vi "DAQ- Steper 2.vi"(0 "Travel (Degree)":dbl=100.0, 5 "Mode":i32(ring)=10178 items=["Finite Samples"=10178, "Continuous Samples"=10123, "Hardware Timed Single Point"=12522], 7 "Home Done":bool, 9 "Speed d/s":dbl=10.0, 11 "error in":errorcluster) -> (6 "Task Done Bit":bool, 15 "error out":errorcluster)   [LabVIEW 2015]
uses:
  Project Setup/Globle Variable/GR_Servo.vi
  <vilib>/DAQmx/create/channels.llb/DAQmx Create Channel (CO-Pulse Generation-Frequency).vi
  <vilib>/DAQmx/configure/timing.llb/DAQmx Timing (Implicit).vi
  Galobal variable_TI.vi
panel:
  out "32bit integer":i32
  in  "Motor PPR":dbl=3600.0
  in  "Motor Gear Ratio":dbl=1.0
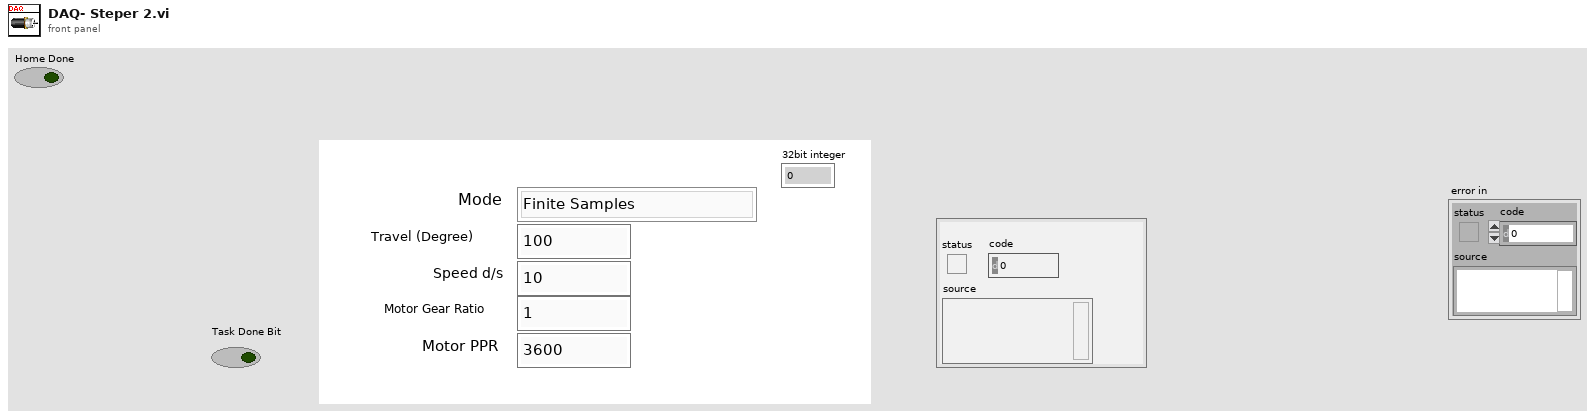
[diagram p1: front panel]
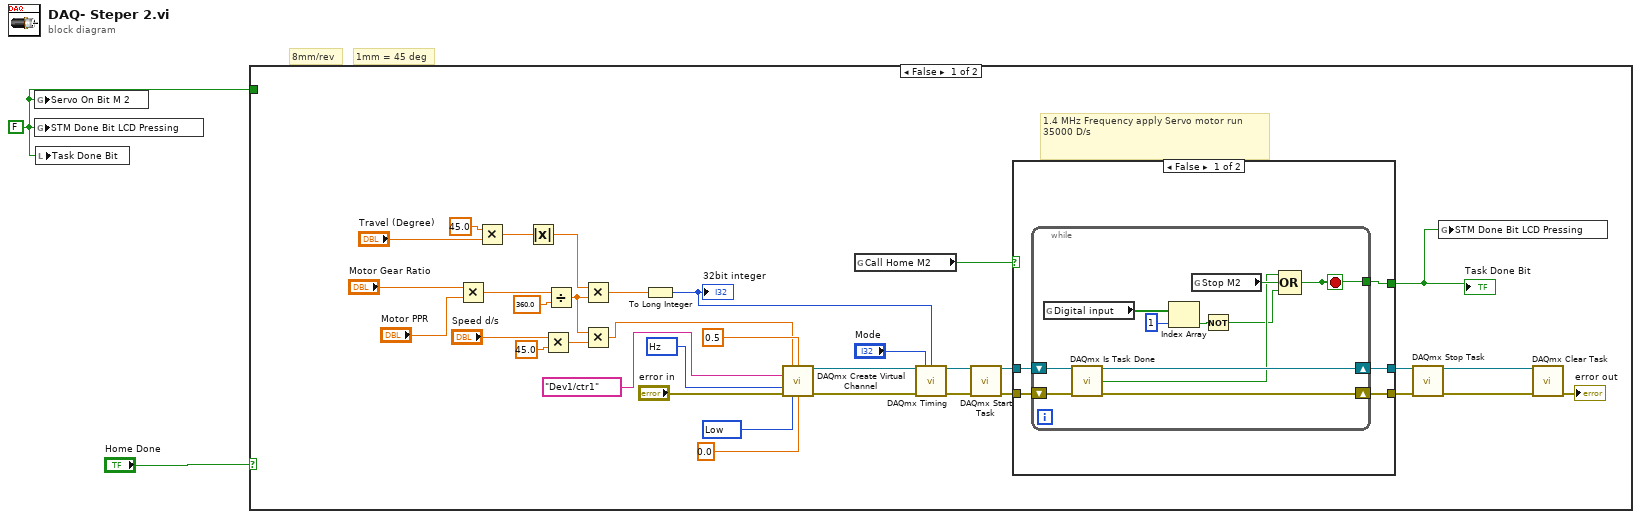
[diagram p0: block diagram]
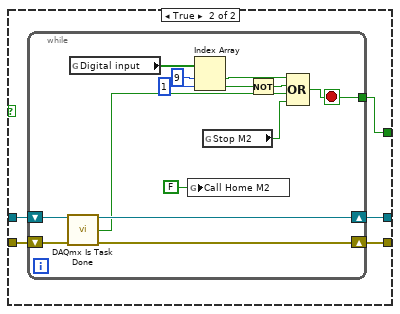
[diagram p2: hidden frame]
diagram:
  w2 = FALSE ("Servo On Bit M 2")
  # "1mm = 45 deg"
  # "8mm/rev"
  n1 = global write "GR_Servo.vi" "Servo On Bit M 2"(w2) -> ()
  n2 = global write "GR_Servo.vi" "STM Done Bit LCD Pressing"(w2) -> ()
  n3 = local write "Task Done Bit"(w2) -> ()
  n4 = case shown="False" "Home Done" {
    tunnel: w2 -> [_ _]
    frame False {
      w16 = 10373 items=["Hz"=10373] ("units")
      w17 = 10214 items=["High"=10192, "Low"=10214] ("idle state")
      # "1.4 MHz Frequency apply Servo motor run \n35000 D/s"
      n5 = Multiply(x="Motor Gear Ratio", y="Motor PPR") -> (x*y=w26:dbl)
      n6 = Multiply(x=45.0, y="Travel (Degree)") -> (x*y=w14:dbl)
      n7 = Absolute Value(x=w14) -> (abs(x)=w25:dbl)
      n8 = Multiply(x="Speed d/s", y=45.0) -> (x*y=w11:dbl)
      n9 = Divide(x=w26, y=360.0) -> (x/y=w30:dbl)
      n10 = Multiply(x=w25, y=w30) -> (x*y=w15:dbl)
      n11 = Multiply(x=w30, y=w11) -> (x*y=w34:dbl)
      n12 = To Long Integer(number=w15) -> (32bit integer=w37:i32)
      "32bit integer" <- w37
      n13 = call-poly <vilib>:"DAQmx Create Virtual Channel.vi"("frequency"=w34, "duty cycle"=0.5, "counter"=tag "Dev1/ctr1", "units"=w16, "error in"="error in", "idle state"=w17, "initial delay"=0.0) -> ("task out"=w19:refnum<k21>, "error out"=w20:errorcluster)  [unwired: 7 in]
      n14 = global read "Galobal variable_TI.vi" "Call Home M2"() -> (w6:bool)
      n15 = call-poly <vilib>:"DAQmx Timing.vi"("task/channels in"=w19, "sample mode"="Mode", "samples per channel"=w37, "error in"=w20) -> ("task out"=w21:refnum<k21>, "error out"=w22:errorcluster)  [unwired: 10 in]
      n16 = call <vilib>:"DAQmx Start Task.vi"("task/channels in"=w21, "error in"=w22) -> ("task out"=w8:refnum<k21>, "error out"=w7:errorcluster)  [unwired: 12 in]
      n17 = case shown="False" w6 {
        tunnel: [w42 w55] -> w4
        tunnel: w8 -> [w41 w58]
        tunnel: [w40 w56] -> w5
        tunnel: w7 -> [w39 w57]
        tunnel: [w38 w54] -> w3
        frame False {
          n18 = while {
            shift-right: [w51] -> w40
            shift-left: w41 -> [w53]
            shift-right: [w52] -> w42
            shift-left: w39 -> [w50]
            tunnel: [w47] -> w38
            stop <- w47 stop-if-true
            n19 = global read "Galobal variable_TI.vi" "Digital input"() -> (w46:bool[])
            n20 = call <vilib>:"DAQmx Is Task Done.vi"("task/channels in"=w53, "error in"=w50) -> ("task out"=w51:refnum<k21>, "task done?"=w48:bool, "error out"=w52:errorcluster)  [unwired: 11 in]
            n21 = Index Array(array=w46, index=1) -> (element=w44:bool)
            n22 = global read "Galobal variable_TI.vi" "Stop M2"() -> (w49:bool)
            n23 = Not(x=w44) -> (.not. x?=w43:bool)
            n24 = Compound Arithmetic op=OR(w48, w49, w43) -> (w47:bool)
          }
        }
        frame True {
          n25 = while {
            shift-right: [w70] -> w56
            shift-left: w58 -> [w72]
            shift-right: [w71] -> w55
            shift-left: w57 -> [w69]
            tunnel: [w64] -> w54
            stop <- w64 stop-if-true
            n26 = call <vilib>:"DAQmx Is Task Done.vi"("task/channels in"=w72, "error in"=w69) -> ("task out"=w70:refnum<k21>, "task done?"=w65:bool, "error out"=w71:errorcluster)  [unwired: 11 in]
            n27 = global read "Galobal variable_TI.vi" "Digital input"() -> (w66:bool[])
            n28 = global write "Galobal variable_TI.vi" "Call Home M2"(FALSE ("Call Home M2")) -> ()
            n29 = Index Array(array=w66, index #1=9 ("index"), index #2=1 ("index")) -> (element #1=w61:bool, element #2=w60:bool)
            n30 = global read "Galobal variable_TI.vi" "Stop M2"() -> (w68:bool)
            n31 = Not(x=w60) -> (.not. x?=w59:bool)
            n32 = Compound Arithmetic op=OR(w61, w59, w65, w68) -> (w64:bool)
          }
        }
      }
      "Task Done Bit" <- w3
      n33 = call <vilib>:"DAQmx Stop Task.vi"("task/channels in"=w5, "error in"=w4) -> ("task out"=w23:refnum<k21>, "error out"=w33:errorcluster)  [unwired: 12 in]
      n34 = global write "GR_Servo.vi" "STM Done Bit LCD Pressing"(w3) -> ()
      n35 = call <vilib>:"DAQmx Clear Task.vi"("task in"=w23, "error in"=w33) -> ("error out"=→"error out":errorcluster)  [unwired: 13 in]
    }
    frame True {
    }
  }
